vi "get AlarmList.vi"(8 "error in (no error)":errorcluster, 11 "map out":T2) -> (0 "error out":errorcluster, 3 "alarm":T1)   [LabVIEW 2022 SP3, in "Alarm interface.lvlib"]
uses:
  Alarm interface.lvlib
  <vilib>/addons/database/_DB Variant To Data/Database Variant To Data.xnode
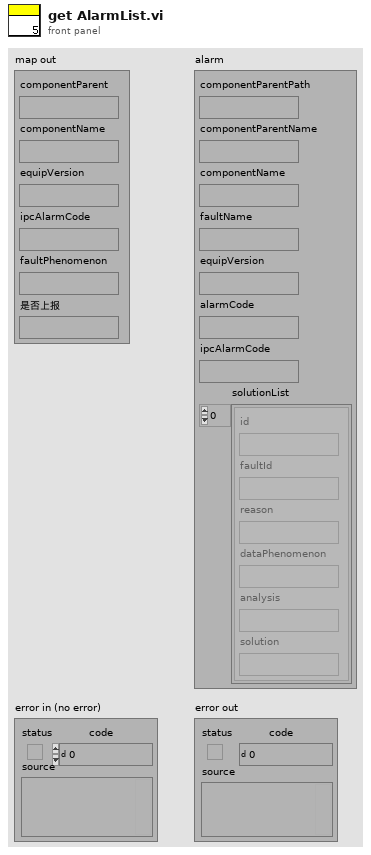
[diagram p1: front panel]
types:
  T1 = cluster{"componentParentPath":string, "componentParentName":string, "componentName":string, "faultName":string, "equipVersion":string, "alarmCode":string, "ipcAlarmCode":string, "solutionList":cluster{"id":string, "faultId":string, "reason":string, "dataPhenomenon":string, "analysis":string, "solution":string}[]}
  T2 = typedef "Alarm interface.lvlib/map out.ctl" = cluster{"componentParent":string, "componentName":string, "equipVersion":string, "ipcAlarmCode":string, "faultPhenomenon":string, "是否上报":string}
  T3 = cluster{"id":string, "faultId":string, "reason":string, "dataPhenomenon":string, "analysis":string, "solution":string}
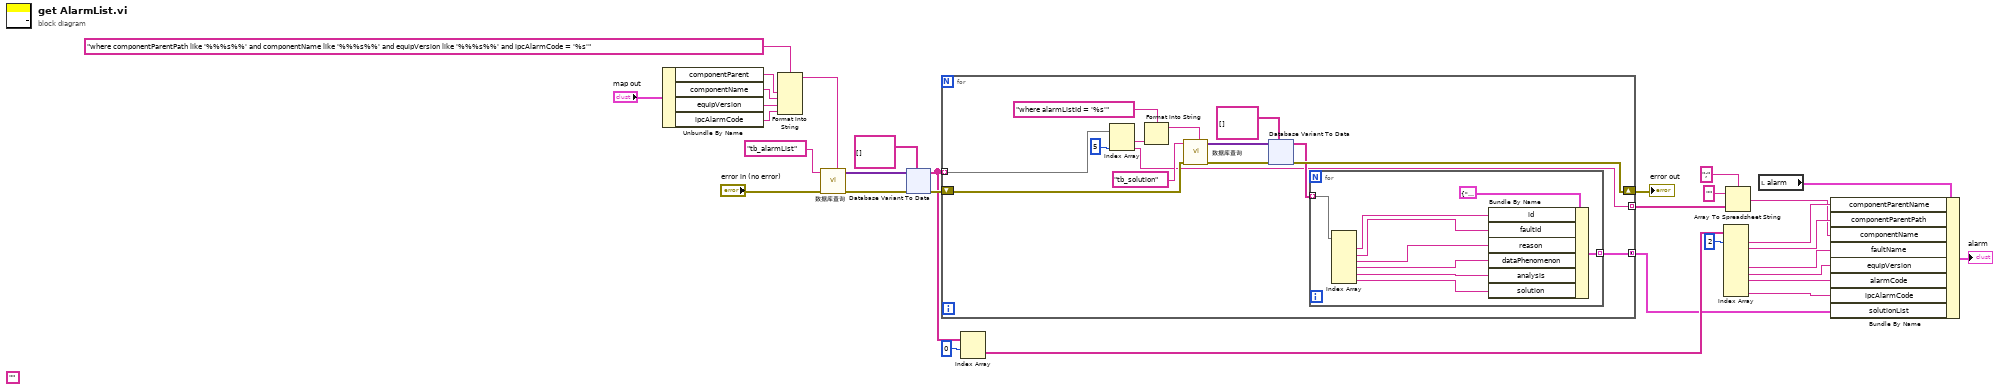
[diagram p0: block diagram]
diagram:
  (unwired) ""
  n1 = Unbundle By Name("map out") -> ("componentParent"=w27:string, "componentName"=w26:string, "equipVersion"=w25:string, "ipcAlarmCode"=w24:string)
  n2 = Format Into String(format string="where componentParentPath like '%%%s%%' and componentName like '%%%s%%' and equipVersion like '%%%s%%' and ipcAlarmCode = '%s'" ("格式字符串"), w27, w26, w25, w24) -> (resulting string=w23:string)  [unwired: 2 in, 1 out]
  n3 = call "数据库查询.vi"("condition"=w23, "error in (no error)"="error in (no error)", "table"="tb_alarmList") -> ("error out"=w18:errorcluster, "data"=w22:variant[][])  [unwired: 6 in, 1 out]
  n4 = xnode "Database Variant To Data"("database variant"=w22, "error in (no error)"=w18, "type"=string[][] []) -> ("data"=w5:string[][], "error out"=w17:errorcluster)
  n5 = for {
    tunnel: [w37] -> w7 mode=concatenating
    shift-right: [w40] -> w16
    shift-left: w17 -> [w45]
    tunnel: w5 -> [w35] mode=indexing
    tunnel: [w32] -> w4 mode=indexing
    n6 = Index Array(array=w35, index #2=5 ("索引")) -> (element #1=w34:string, element #2=w32:string)  [unwired: 1 in]
    n7 = Format Into String(format string="where alarmListId = '%s'" ("格式字符串"), w34) -> (resulting string=w43:string)  [unwired: 2 in, 1 out]
    n8 = call "数据库查询.vi"("condition"=w43, "error in (no error)"=w45, "table"="tb_solution") -> ("error out"=w41:errorcluster, "data"=w42:variant[][])  [unwired: 6 in, 1 out]
    n9 = xnode "Database Variant To Data"("database variant"=w42, "error in (no error)"=w41, "type"=string[][] []) -> ("data"=w38:string[][], "error out"=w40:errorcluster)
    n10 = for {
      tunnel: w38 -> [w53] mode=indexing
      tunnel: [w48] -> w37 mode=indexing
      n11 = Index Array(array=w53) -> (element #1=w52:string, element #2=w51:string, element #3=w46:string, element #4=w50:string, element #5=w47:string, element #6=w49:string)  [unwired: 6 in]
      n12 = Bundle By Name(cluster=T3 {"id"="", "faultId"="", "reason"="", "dataPhenomenon"="", "analysis"="", "solution"=""} ("solutionList"), "id"=w52, "faultId"=w51, "reason"=w46, "dataPhenomenon"=w50, "analysis"=w47, "solution"=w49) -> (w48:T3)
    }
  }
  "error out" <- w16
  n13 = Index Array(array=w5, index (row)=0 ("索引 (行)")) -> (element=w19:string[])  [unwired: 1 in]
  n14 = Index Array(array=w19, index #1=2 ("索引")) -> (element #1=w13:string, element #2=w12:string, element #5=w11:string, element #6=w10:string, element #7=w9:string, element #9=w8:string)  [unwired: 8 in, 3 out]
  n15 = Array To Spreadsheet String(delimiter (Tab)=";" ("分隔符(Tab)"), array=w4, 3:"" ("格式字符串")) -> (spreadsheet string=w2:string)
  n16 = local read "alarm"() -> (w15:T1)
  n17 = Bundle By Name(cluster=w15, "componentParentName"=w13, "componentParentPath"=w12, "componentName"=w2, "faultName"=w11, "equipVersion"=w10, "alarmCode"=w9, "ipcAlarmCode"=w8, "solutionList"=w7) -> (→"alarm":T1)
